vi "Event Handler.vi"(8 "error in (no error)":errorcluster, 10 "Stop Event Handler":refnum<user-event>, 11 "ColorSelector in":refnum<class "ColorSelector.lvclass">) -> (0 "error out":errorcluster)   [LabVIEW 2015, in "ColorSelector.lvclass"]
doc: "The <b>Event Handler VI</b> is a dynamic dispatch VI that should be overwritten if events are needed to create the enhanced QControl. \n\nBy inheriting from the main Control.lvclass the overwritten <b>Event Handler VI</b> will be launched asynchronously in the initialization of the QControl.\n<b> </b> <b> </b>\n©2017 Q Software Innovations, LLC (QSI)\nwritten by Quentin Alldredge\nproduced in LabVIEW 2015\n\nsupport@qsoftwareinnovations.com\nwww.qsoftwareinnovations.com\n\nAll rights reserved.\n\nRedistribution and use in source and binary forms, with or without modification, are permitted provided that the following conditions are met:\n\n * Redistributions of source code must retain the above copyright notice, this list of conditions and the following disclaimer.\n * Redistributions in binary form must reproduce the above copyright notice, this list of conditions and the following disclaimer in the documentation and/or other materials provided with the distribution.\n * Neither the name of Q Software Innovations, LLC. nor the names of its contributors may be used to endorse or promote products derived from this software without specific prior written permission.\n\nTHIS SOFTWARE IS PROVIDED BY THE COPYRIGHT HOLDERS AND CONTRIBUTORS \"AS IS\" AND ANY EXPRESS OR IMPLIED WARRANTIES, INCLUDING, BUT NOT LIMITED TO, THE IMPLIED WARRANTIES OF MERCHANTABILITY AND FITNESS FOR A PARTICULAR PURPOSE ARE DISCLAIMED. IN NO EVENT SHALL THE COPYRIGHT OWNER OR CONTRIBUTORS BE LIABLE FOR ANY DIRECT, INDIRECT, INCIDENTAL, SPECIAL, EXEMPLARY, OR CONSEQUENTIAL DAMAGES (INCLUDING, BUT NOT LIMITED TO, PROCUREMENT OF SUBSTITUTE GOODS OR SERVICES; LOSS OF USE, DATA, OR PROFITS; OR BUSINESS INTERRUPTION) HOWEVER CAUSED AND ON ANY THEORY OF LIABILITY, WHETHER IN CONTRACT, STRICT LIABILITY, OR TORT (INCLUDING NEGLIGENCE OR OTHERWISE) ARISING IN ANY WAY OUT OF THE USE OF THIS SOFTWARE, EVEN IF ADVISED OF THE POSSIBILITY OF SUCH DAMAGE."
uses:
  ColorSelector.lvclass
  ColorSelector.lvclass/ColorSelector.ctl
  Active Selector Enum.ctl
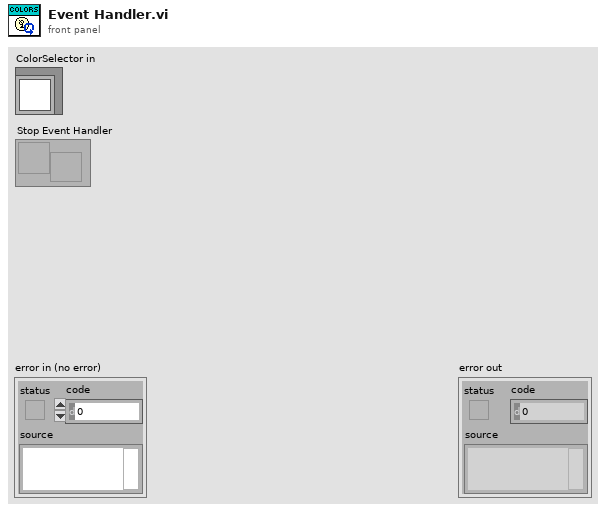
[diagram p1: front panel]
types:
  T1 = typedef "ColorSelector.lvclass/Active Selector Enum.ctl" = enum16{"Grey", "Color"}
  T2 = typedef "LVPoint32TypeDef.ctl" = cluster{"Horizontal":i32, "Vertical":i32}
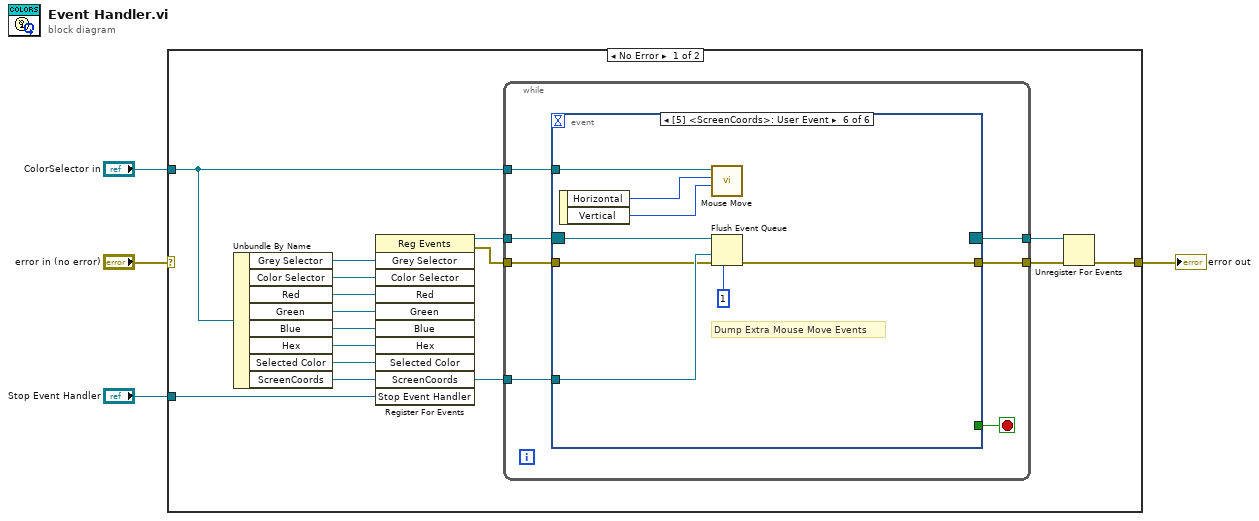
[diagram p0: block diagram]
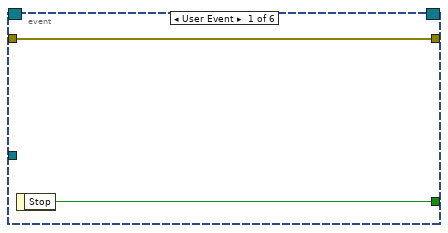
[diagram p2: hidden frame]
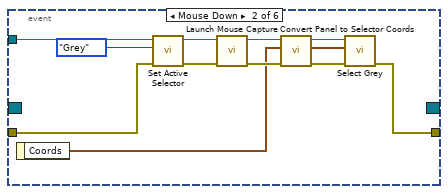
[diagram p3: hidden frame]
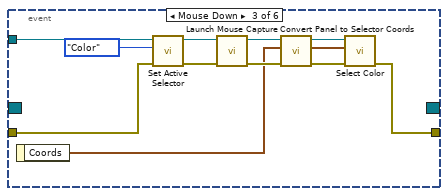
[diagram p4: hidden frame]
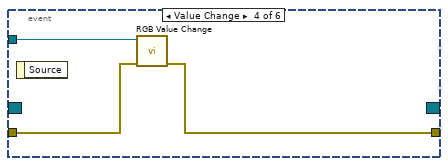
[diagram p5: hidden frame]
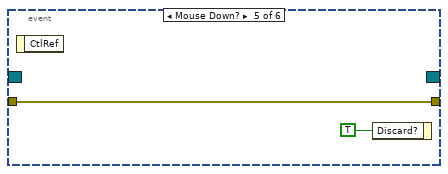
[diagram p6: hidden frame]
diagram:
  n1 = case shown="No Error" "error in (no error)" {
    selector: "error in (no error)" -> [_ w66]
    tunnel: [w18 w66] -> w3
    tunnel: "ColorSelector in" -> [w16 _]
    tunnel: "Stop Event Handler" -> [w15 _]
    frame No Error {
      n2 = Unbundle By Name(w16) -> ("Grey Selector"=w14:refnum<vi>, "Color Selector"=w13:refnum<vi>, "Red"=w9:refnum<vi>, "Green"=w8:refnum<vi>, "Blue"=w7:refnum<vi>, "Hex"=w5:refnum<vi>, "Selected Color"=w6:refnum<vi>, "ScreenCoords"=w11:refnum<user-event>)
      n3 = register-events(w14, w13, w9, w8, w7, w5, w6, w11, w15) -> (reference out=w10:refnum<event-registration>, error out=w12:errorcluster)  [unwired: 2 in]
      n4 = while {
        tunnel: w10 -> [w26]
        tunnel: w12 -> [w24]
        tunnel: [w23] -> w19
        tunnel: [w21] -> w17
        tunnel: w16 -> [w25]
        tunnel: w11 -> [w20]
        stop <- w22 stop-if-true
        n5 = event shown="[5] <ScreenCoords>: User Event" {
          selector: w26 -> [_ _ _ _ _ w62]
          dyn-events: [_ _ _ _ _ _] -> w21
          timeout: _ -> [_ _ _ _ _ _]
          tunnel: w25 -> [_ w40 w50 w55 _ w65]
          tunnel: w24 -> [w28 w35 w48 w54 w56 w59]
          tunnel: [w28 w36 w47 w53 w56 w58] -> w23
          tunnel: [w27 _ _ _ _ _] -> w22
          tunnel: w20 -> [_ _ _ _ _ w61]
          event User Event {
            n6 = event-data() -> ("Stop"=w27:bool)  [unwired: 1 in]
          }
          event Mouse Down {
            n7 = event-data() -> ("Coords"=w32:T2)  [unwired: 1 in]
            n8 = call "Set Active Selector.vi"("error in (no error)"=w35, "ActiveSelector"=Active_Selector_Enum."Grey", "ColorSelector in"=w40) -> ("error out"=w37:errorcluster, "ColorSelector out"=w39:refnum<class "ColorSelector.lvclass">)  [unwired: 7 in]
            n9 = call "Launch Mouse Capture.vi"("error in (no error)"=w37, "ColorSelector in"=w39) -> ("error out"=w33:errorcluster, "ColorSelector (dup)"=w34:refnum<class "ColorSelector.lvclass">)  [unwired: 8 in]
            n10 = call "Convert Panel to Selector Coords.vi"("error in (no error)"=w33, "Coords in (Panel)"=w32, "ColorSelector in"=w34) -> ("error out"=w29:errorcluster, "Coords in (Control)"=w31:T2, "ColorSelector (dup)"=w30:refnum<class "ColorSelector.lvclass">)  [unwired: 6 in]
            n11 = call "Select Grey.vi"("error in (no error)"=w29, "Coords"=w31, "ColorSelector in"=w30) -> ("error out"=w36:errorcluster)  [unwired: 7 in, 1 out]
          }
          event Mouse Down {
            n12 = event-data() -> ("Coords"=w42:T2)  [unwired: 1 in]
            n13 = call "Set Active Selector.vi"("error in (no error)"=w48, "ActiveSelector"=Active_Selector_Enum."Color", "ColorSelector in"=w50) -> ("error out"=w49:errorcluster, "ColorSelector out"=w51:refnum<class "ColorSelector.lvclass">)  [unwired: 7 in]
            n14 = call "Launch Mouse Capture.vi"("error in (no error)"=w49, "ColorSelector in"=w51) -> ("error out"=w44:errorcluster, "ColorSelector (dup)"=w46:refnum<class "ColorSelector.lvclass">)  [unwired: 8 in]
            n15 = call "Convert Panel to Selector Coords.vi"("error in (no error)"=w44, "Coords in (Panel)"=w42, "ColorSelector in"=w46) -> ("error out"=w43:errorcluster, "Coords in (Control)"=w41:T2, "ColorSelector (dup)"=w45:refnum<class "ColorSelector.lvclass">)  [unwired: 6 in]
            n16 = call "Select Color.vi"("error in (no error)"=w43, "Coords in"=w41, "ColorSelector in"=w45) -> ("error out"=w47:errorcluster)  [unwired: 7 in, 1 out]
          }
          event Value Change {
            n17 = event-data() -> ()  [unwired: 1 in, 1 out]
            n18 = call "RGB Value Change.vi"("error in (no error)"=w54, "ColorSelector in"=w55) -> ("error out"=w53:errorcluster)  [unwired: 8 in, 1 out]
          }
          event Mouse Down? {
            n19 = event-data() -> ()  [unwired: 1 in, 1 out]
            n20 = event-data("Discard?"=TRUE) -> ()  [unwired: 1 in, 1 out]
          }
          event User Event {
            # "Dump Extra Mouse Move Events"
            n21 = event-data() -> ("Horizontal"=w64:i32, "Vertical"=w63:i32)  [unwired: 1 in]
            n22 = call "Mouse Move.vi"("Vertical"=w63, "Horizontal"=w64, "ColorSelector in"=w65) -> ()  [unwired: 7 in, 2 out]
            n23 = Flush Event Queue(0:w62, 2:w61, 3:w59, 5:1 ("keep most recent")) -> (11:w58:errorcluster)  [unwired: 2 in, 2 out]
          }
        }
      }
      n24 = Unregister For Events(event registration refnum=w17, error in=w19) -> (error out=w18:errorcluster)
    }
    frame Error {
    }
  }
  "error out" <- w3
